vi "upload_session_finish.vi"(8 "error in (no error)":errorcluster, 9 "path":string, 10 "offset":i64, 11 "session_id":string) -> (0 "error out":errorcluster)   [LabVIEW 2015, in "lv-dropbox.lvlib" / "v2.lvlib"]
uses:
  v2.lvlib
  private/_controls/content_type.ctl
  <vilib>/httpClient/POSTBuffer.vi
  lv-dropbox.lvlib
  <vilib>/httpClient/LabVIEWHTTPClient.lvlib
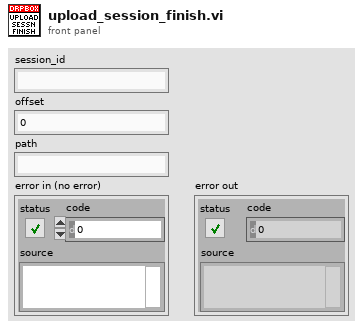
[diagram p1: front panel]
types:
  T1 = cluster{"cursor":cluster{"session_id":string, "offset":i64}, "commit":cluster{"path":string}}
  T2 = typedef "lv-dropbox.lvlib/content_type.ctl" = enum16{"<content_type>", "application/json", "application/octet-stream", "application/x-www-form-urlencoded"}
  T3 = cluster{"name":string, "path_lower":string, "id":string, "client_modified":string, "server_modified":string, "rev":string, "size":u64}
  T4 = typedef "LabVIEWHTTPClient.lvlib/ClientHandle.ctl" = refnum<k1>
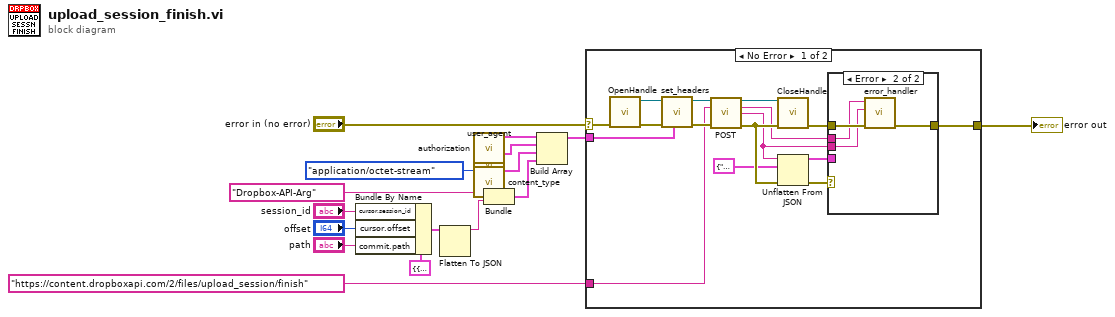
[diagram p0: block diagram]
diagram:
  n1 = Bundle By Name(cluster=T1 {"cursor"={"session_id"="", "offset"=0}, "commit"={"path"=""}}, "cursor.session_id"="session_id", "cursor.offset"="offset", "commit.path"="path") -> (w7:T1)
  n2 = Flatten To JSON(anything=w7) -> (JSON string=w6:string)  [unwired: 2 in, 1 out]
  n3 = call "authorization.vi"() -> ("header"=w12:cluster{"header":string, "value":string})  [unwired: 11 in]
  n4 = call "user_agent.vi"() -> ("header"=w15:cluster{"header":string, "value":string})  [unwired: 11 in]
  n5 = call "content_type.vi"("content_type"=content_type."application/octet-stream") -> ("header"=w16:cluster{"header":string, "value":string})  [unwired: 10 in]
  n6 = Bundle("header"="Dropbox-API-Arg", "JSON string"=w6) -> (w2:cluster{"header":string, "JSON string":string})  [unwired: 1 in]
  n7 = Build Array(w12, w15, w16, w2) -> (w11:cluster{"header":string, "JSON string":string}[])
  n8 = case shown="No Error" "error in (no error)" {
    selector: "error in (no error)" -> [w27 w38]
    tunnel: w11 -> [w26 _]
    tunnel: "https://content.dropboxapi.com/2/files/upload_session/finish" ("url") -> [w25 _]
    tunnel: [w21 w38] -> w10
    frame No Error {
      n9 = call <vilib>:"OpenHandle.vi"("error in (no error)"=w27) -> ("client handle out"=w30:T4, "error out"=w23:errorcluster)  [unwired: 13 in]
      n10 = call "set_headers.vi"("header_value []"=w26, "error in (no error)"=w23, "client_handle in"=w30) -> ("error out"=w28:errorcluster, "client_handle out"=w29:T4)  [unwired: 7 in]
      n11 = call-poly <vilib>:"POST.vi"("client handle"=w29, "url"=w25, "error in (no error)"=w28) -> ("client handle out"=w31:T4, "headers"=w19:string, "body"=w20:string, "error out"=w32:errorcluster)  [unwired: 9 in]
      n12 = call <vilib>:"CloseHandle.vi"("client handle"=w31, "error in (no error)"=w32) -> ("error out"=w22:errorcluster)  [unwired: 13 in]
      n13 = Unflatten From JSON(JSON string=w20, type and defaults=T3 {"name"="", "path_lower"="", "id"="", "client_modified"="", "server_modified"="", "rev"="", "size"=0}, error in (no error)=w32) -> (value=w17:T3, error out=w18:errorcluster)  [unwired: 4 in]
      n14 = case shown="Error" w18 {
        tunnel: w19 -> [_ w36]
        tunnel: w20 -> [_ w35]
        tunnel: [w33 w34] -> w21
        tunnel: w22 -> [w33 w37]
        tunnel: w17 -> [_ _]
        frame No Error {
        }
        frame Error {
          n15 = call "error_handler.vi"("error in (no error)"=w37, "body"=w35, "headers"=w36) -> ("error out"=w34:errorcluster)  [unwired: 8 in]
        }
      }
    }
    frame Error {
    }
  }
  "error out" <- w10
